vi "2D Convolution (CDB).vi"(8 "output size":enum32{"full", "size X", "compact"}(ring), 9 "algorithm":enum32{"direct", "frequency domain"}(ring)=enum."frequency domain", 10 "Y":cdb[][](array[numeric]), 11 "X":cdb[][](array[numeric])) -> (0 "error":i32, 3 "X * Y":cdb[][](array[numeric]))   [LabVIEW 2010, in "NI_AALPro.lvlib"]
doc: "Computes the convolution of the input sequences <B>X</B> and <B>Y</B>. Wire data to the <B>X</B> input to determine the polymorphic instance to use or manually select the instance."
uses:
  NI_AALPro.lvlib
  lvanlys.dll
panel:
  # "2D Convolution (CDB)"
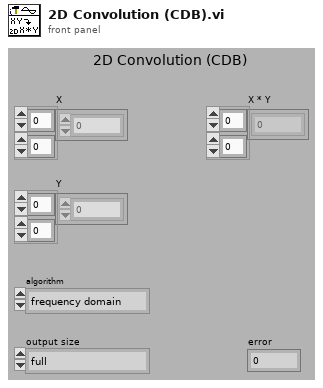
[diagram p1: front panel]
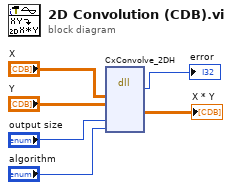
[diagram p0: block diagram]
diagram:
  n1 = dll-call lib="C:/Program Files/National Instruments/LabVIEW 2010/resource/lvanlys.*" fn="CxConvolve_2DH"("X"="X", "Y"="Y", "size"="output size", "domain"="algorithm") -> (→"error":i32, "X * Y"=→"X * Y":cdb[][])  [unwired: 8 in, 2 out]
